vi "niDTS WLAN OFDM Tx Test UTIL WLAN to OFDM ModAcc Settings.vi"(10 "ModAcc Measurement Paramaters":T2={"ModAcc Enable"=FALSE, "Header Detection"=enum."FIRST", "Averages"=3, "Amplitude Tracking"=FALSE, "Channel Tracking"=FALSE, "Time Tracking"=TRUE, "Phase Tracking"=enum."NONE", "Clock Offset Est"=FALSE, "Impairments Est"=FALSE, "CFO Estimation"=enum."PAMBLE"}) -> (2 "OFDM ModAcc Measurement Paramaters":T1={"ModAcc Enable"=FALSE, "Header Detection"=enum."FIRST", "Averages"=0, "CFO Estimation"=enum."PAMBLE", "Amplitude Tracking"=FALSE, "Channel Tracking"=FALSE, "Time Tracking"=FALSE, "Phase Tracking"=enum."NONE", "Clock Offset Est"=FALSE, "Impairments Est"=FALSE})   [LabVIEW 2015, in "niDTS WLAN.lvlib"]
uses:
  niDTS WLAN.lvlib
  Includes/niDTS WLAN INC ModAcc Measurement Parameters.ctl
  Includes/niDTS WLAN OFDM Tx Test INC ModAcc Measurement Parameters.ctl
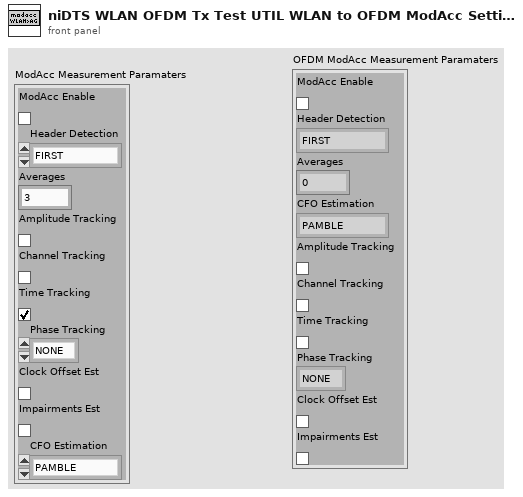
[diagram p1: front panel]
types:
  T1 = typedef "niDTS WLAN.lvlib/niDTS WLAN OFDM Tx Test INC ModAcc Measurement Parameters.ctl" = cluster{"ModAcc Enable":bool, "Header Detection":enum16{"MANUAL", "FIRST", "ALL"}, "Averages":i32, "CFO Estimation":enum16{"PAMBLE", "PDATA"}, "Amplitude Tracking":bool, "Channel Tracking":bool, "Time Tracking":bool, "Phase Tracking":enum16{"NONE", "STANDARD", "CSF", "INSTANT"}, "Clock Offset Est":bool, "Impairments Est":bool}
  T2 = typedef "niDTS WLAN.lvlib/niDTS WLAN INC ModAcc Measurement Parameters.ctl" = cluster{"ModAcc Enable":bool, "Header Detection":enum16{"MANUAL", "FIRST", "ALL"}, "Averages":i32, "Amplitude Tracking":bool, "Channel Tracking":bool, "Time Tracking":bool, "Phase Tracking":enum16{"NONE", "STANDARD", "CSF", "INSTANT"}, "Clock Offset Est":bool, "Impairments Est":bool, "CFO Estimation":enum16{"PAMBLE", "PDATA"}}
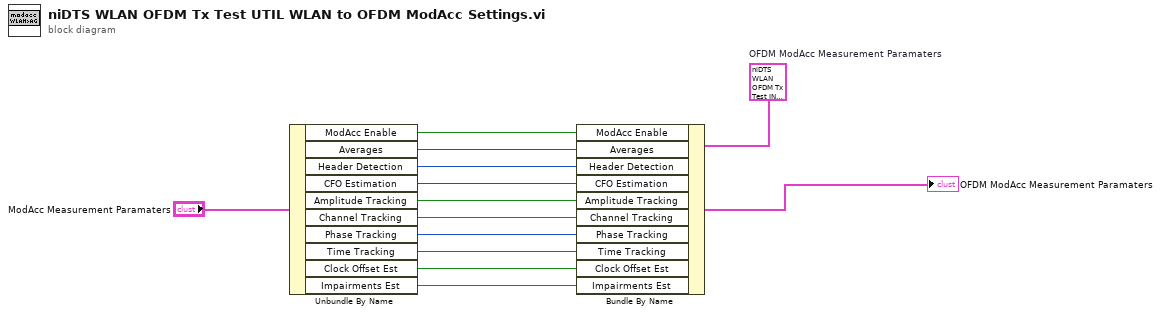
[diagram p0: block diagram]
diagram:
  w6 = T1 {"ModAcc Enable"=FALSE, "Header Detection"=enum."FIRST", "Averages"=0, "CFO Estimation"=enum."PAMBLE", "Amplitude Tracking"=FALSE, "Channel Tracking"=FALSE, "Time Tracking"=FALSE, "Phase Tracking"=enum."NONE", "Clock Offset Est"=FALSE, "Impairments Est"=FALSE}  # OFDM ModAcc Measurement Paramaters
  n1 = Unbundle By Name("ModAcc Measurement Paramaters") -> ("ModAcc Enable"=w4:bool, "Averages"=w13:i32, "Header Detection"=w3:enum16{"MANUAL", "FIRST", "ALL"}, "CFO Estimation"=w12:enum16{"PAMBLE", "PDATA"}, "Amplitude Tracking"=w11:bool, "Channel Tracking"=w10:bool, "Phase Tracking"=w9:enum16{"NONE", "STANDARD", "CSF", "INSTANT"}, "Time Tracking"=w8:bool, "Clock Offset Est"=w2:bool, "Impairments Est"=w1:bool)
  n2 = Bundle By Name(cluster=w6, "ModAcc Enable"=w4, "Averages"=w13, "Header Detection"=w3, "CFO Estimation"=w12, "Amplitude Tracking"=w11, "Channel Tracking"=w10, "Phase Tracking"=w9, "Time Tracking"=w8, "Clock Offset Est"=w2, "Impairments Est"=w1) -> (→"OFDM ModAcc Measurement Paramaters":T1)
